vi "CMI LiB Bias Set Bias.vi"(8 "error in":errorcluster, 9 "channel index (0: first)":i32, 10 "bias [V]":dbl, 11 "VISA in":refnum<visa-resource-name>) -> (0 "error out":errorcluster, 3 "VISA out":refnum<visa-resource-name>)   [LabVIEW 2013]
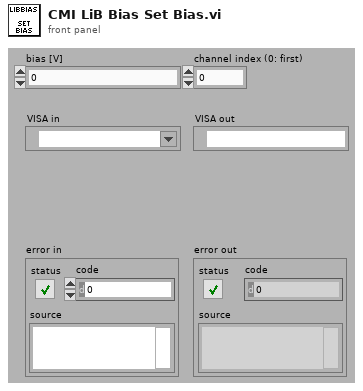
[diagram p1: front panel]
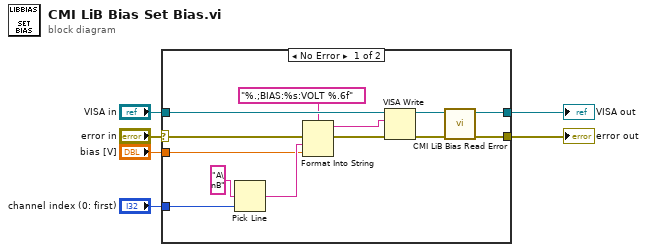
[diagram p0: block diagram]
diagram:
  n1 = case shown="No Error" "error in" {
    selector: "error in" -> [w18 w21]
    tunnel: "VISA in" -> [w17 w20]
    tunnel: [w8 w20] -> w5
    tunnel: [w7 w21] -> w4
    tunnel: "channel index (0: first)" -> [w15 _]
    tunnel: "bias [V]" -> [w12 _]
    frame No Error {
      n2 = Pick Line(multi-line string="A\nB", line index=w15) -> (output string=w13:string)  [unwired: 1 in]
      n3 = Format Into String(format string="%.;BIAS:%s:VOLT %.6f", error in=w18, w13, w12) -> (resulting string=w11:string, error out=w19:errorcluster)  [unwired: 1 in]
      n4 = VISA Write(VISA resource name=w17, write buffer=w11, error in (no error)=w19) -> (VISA resource name out=w9:refnum<visa-resource-name>, error out=w10:errorcluster)  [unwired: 1 out]
      n5 = call "CMI LiB Bias Read Error.vi"("error in"=w10, "VISA in"=w9) -> ("error out"=w7:errorcluster, "VISA out"=w8:refnum<visa-resource-name>)  [unwired: 7 in, 1 out]
    }
    frame Error {
    }
  }
  "error out" <- w4
  "VISA out" <- w5
